vi "Задание_АБ_новые_наработки.vi"() -> ()   [LabVIEW 2017]
uses:
  <vilib>/Analysis/baseanly.llb/Mean (DBL).vi
  <vilib>/gmath/statdist.llb/Beta Random.vi
  <vilib>/Analysis/3filter.llb/Bessel Filter (DBL).vi
  <vilib>/Analysis/NI_AALBase.lvlib
  <vilib>/gmath/NI_Gmath.lvlib
panel:
  out "output array":dbl[](array[numeric])
  out "Array 2":dbl[](array[numeric])
  out "Numeric":i32
  out "Последовательность в массиве":dbl[](array[numeric])
  in  "Кол-во элементов":i32=16
  out "Numeric":dbl
  out "Array":dbl[](array[numeric])
  out "Исходное сообщение":dbl[](array[numeric])
  out "Подготовленный к отправке мажоритарный код":dbl[][](array[numeric])
  out "2-х массив на выходе 3":dbl[][](array[numeric])
  in  "Размер окна":i32=4
  in  "Кол-во копий":i32=5
  out "Шум на основе распределения Рэлея":dbl[](graph)
  out "Итого. кол-во бит":i32
  in  "Пороговое значение":dbl
  out "Демодулированный и отфильтрованный сигнал":dbl[][](graph)
  out "Демодулированный сигнал":i16[](graph)
  in  "Нижняя частота среза":dbl
  in  "Порядок фильтра":i64(slide) scale=0.0..20.0
  in  "Переменная floor(x/y)":i32
  out "Модулирующий сигнал":dbl[](graph)
  out "Частотно модулированный цифровой сигнал":dbl[](graph)
  in  "см. 1.2 Циклов в секунду":i32(slide) scale=4.0..50.0
  in  "Сколько битов брать":i32=4
  out "Радио сигнал с паузами":dbl[](graph)
  in  "Кол-во выборок":i32=400
  out "Массив с паузами":dbl[](array[numeric])
  in  "Количество бит":i32=8
  out "Вырезка из массива":dbl[](array[numeric])
  out "Биты на выходе 1":dbl[](array[numeric])
  # "Демодуляция"
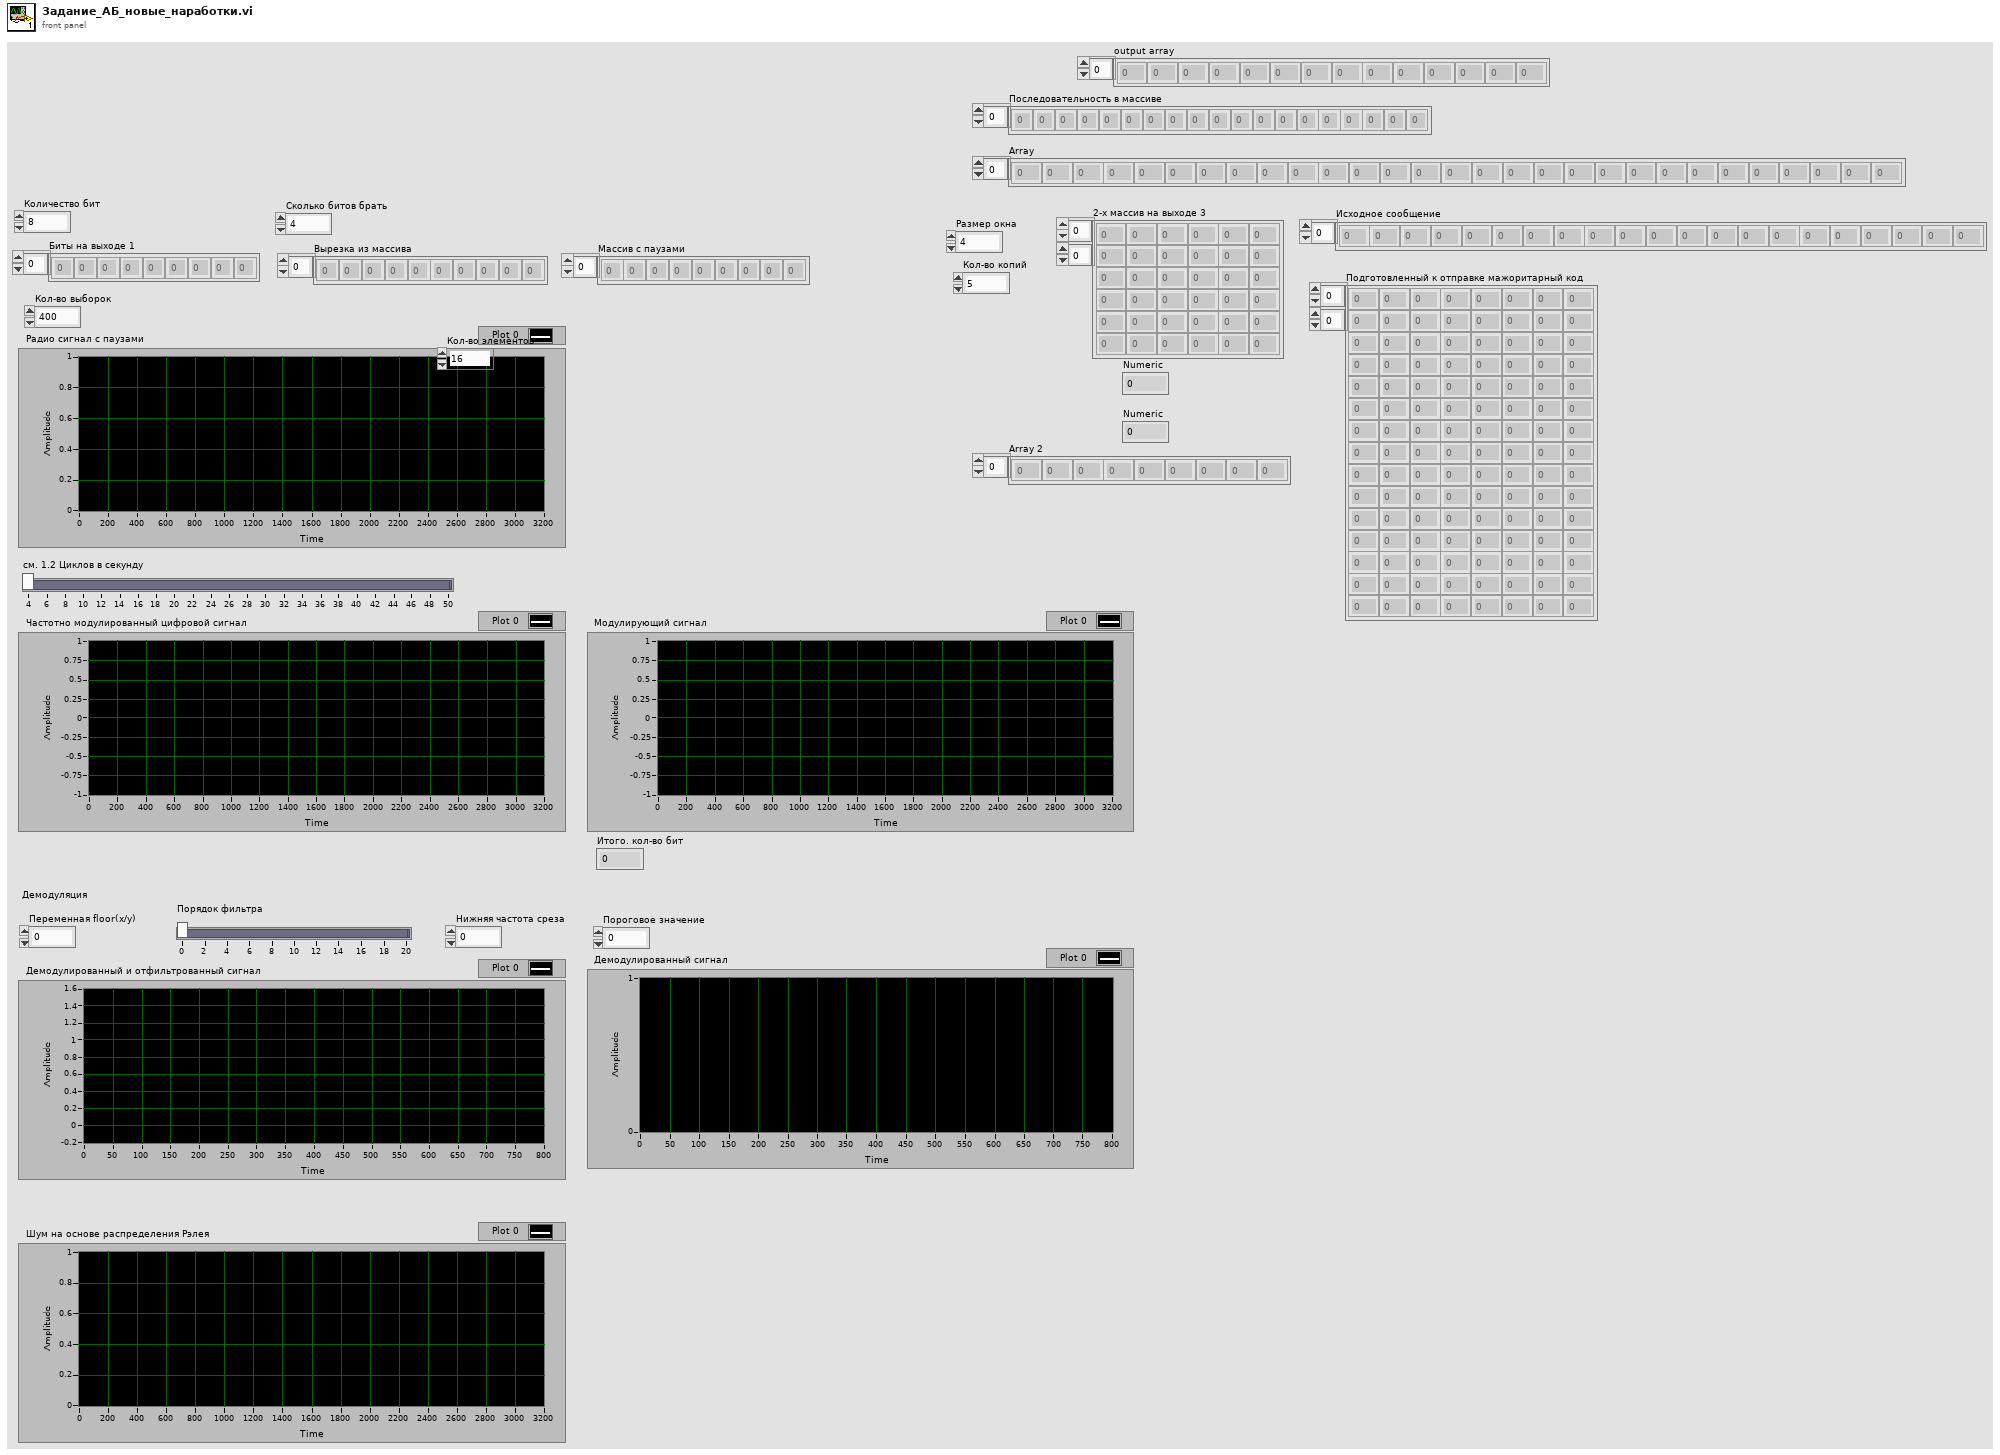
[diagram p1: front panel]
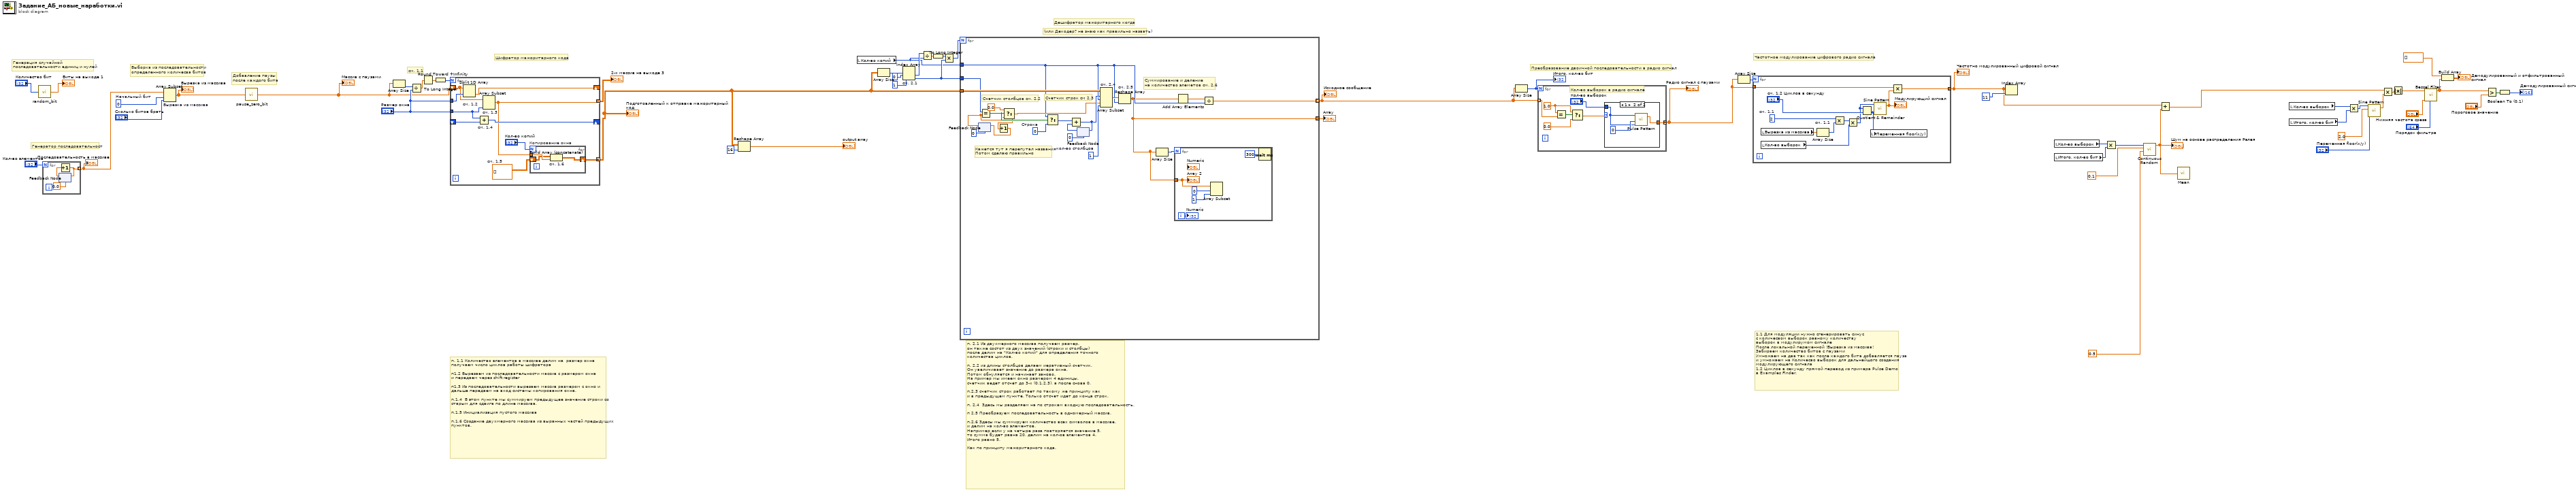
[diagram p0: block diagram]
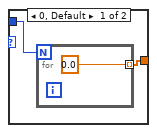
[diagram p2: hidden frame]
diagram:
  w56 = 0  # Начальный бит
  # "Генератор последовательност"
  # "п. 2.1 Из двухмерного массива получаем размер.\nон также состот из двух значений (строки и столбцы) \nпосле делим на \"Кол-во копий\" для определения точного\nколичества циклов.\n\nп. 2.2 из длины столбцов делаем иеративный счетчик. \nОн увеличивает значение до размера окна.\nПотом обнуляется и начинает заново.\nНа пример мы имеем окно размером 4 единицы.\nсчетчик ведет отсчет до 3-х (0,1,2,3), а после снова 0.\n\nп.2.3 счетчик строк работает по такому же принципу как \nи в предыдущем пункте. Только отсчет идет до конца строк.\n\nп. 2.4  Здесь мы разделяем на по строкам входную последовательность.\n\nп 2.5 Преобразуем последовательность в одномерный массив.\n\nп.2.6 Здесы мы суммируем количество всех символов в массиве.\nи делим на кол-во элементов.\nНапример если у на четыре раза повторяется значение 5, \nто сумма будет равна 20, делим на кол-ов элементов 4. \nИтого равно 5. \n\nКак по принципу мажоритарного кода."
  # "см. 1.1"
  # "(или Декодер? не знаю как правильно назвать)"
  # "Дешифратор мажоритарного когда"
  # "п. 1.1 Количество элементов в массиве делим на  размер окна\nполучаем число циклов работы шифратора\n\nп1.2 Вырезаем из последовательности массив с размером окна \nи передаем через shift register\n\nп1.3 Из последовательности вырезаем массив размером с окно и \nдальше передаем на вход системы копирования окна.\n \nп.1.4  В этом пункте мы суммируем предыдущее значение строки со\nстарым для сдвига по длине массива.\n\nп.1.5 Инициализация пустого массива\n\nп.1.6 Создание двухмерного массива из выранных частей предыдущих\nпунктов."
  # "Шифратор мажоритарного кода"
  # "1.1 Для модуляции нужно сгенерировать синус \nс количесвом выборок равному количеству \nвыборок в модулирумом сигнале\nПосле локальной переменной !Вырезка из массива! \nЗабираем количество битов с паузами \nУмножаем на два так как после каждого бита добавляется пауза\nи умножаем на Количесво выборок для дальнейшого создания  \nмодулирующего сигнала\n1.2 Циклов в секунду прямой перевод из примера Pulse Demo \nв Examples Finder."
  # "Преобразование двоичной последовательности в радио сигнал"
  # "Частотное модулирование цифрового радио сигнала"
  # "Добавление паузы \nпосле каждого бита"
  # "Выборка из последовательности\nопределенного количесва битов"
  # "Генерация случайной \nпоследовательности единиц и нулей"
  n1 = call "random_bit.vi"("Количество бит"="Количество бит") -> ("Биты на выходе 1"=→"Биты на выходе 1":dbl[])
  n2 = for {
    N: "Кол-во элементов" -> [_]
    tunnel: [w57] -> w4 mode=indexing
    n3 = feedback #1(0.0) -> (w59:dbl)
    n4 = Increment(x=w59) -> (x+1=w57:dbl)
    n5 = feedback-in #1(w57) -> ()
  }
  "Последовательность в массиве" <- w4
  n6 = Array Subset "Вырезка из массива"(array=w4, index=w56, length="Сколько битов брать") -> (w9:dbl[])
  "Вырезка из массива" <- w9
  n7 = call "pause_zero_bit.vi"("Входная последовательность"=w9) -> ("Массив с паузами"=w8:dbl[])
  "Массив с паузами" <- w8
  n8 = Array Size(array=w8) -> (size(s)=w26:i32)
  n9 = Divide(x=w26, y="Размер окна") -> (x/y=w25:dbl)
  n10 = Round Toward +Infinity(x=w25) -> (ceil(x): smallest int >= x=w24:dbl)
  n11 = To Long Integer(number=w24) -> (32bit integer=w21:i32)
  n12 = for {
    N: w21 -> [_]
    shift-right: [w69] -> _
    shift-left: w8 -> [w67]
    tunnel: "Размер окна" -> [w68]
    shift-right: [w65] -> _
    shift-left: _ -> [w64]
    tunnel: "Размер окна" -> [w66]
    tunnel: [w62] -> w22 mode=indexing
    tunnel: [w61] -> w3 mode=concatenating
    w60 = dbl[][] []  # см. 1.5
    n13 = Split 1D Array "см. 1.2"(array=w67, index=w68) -> (second subarray=w69:dbl[])  [unwired: 1 out]
    n14 = Add "см. 1.4"(x=w66, y=w64) -> (x+y=w65:i32)
    n15 = Array Subset "см. 1.3"(array=w67, length=w66) -> (w62:dbl[])  [unwired: 1 in]
    n16 = for "Копирование окна" {
      N: "Кол-во копий" -> [_]
      tunnel: w62 -> [w71]
      shift-right: [w72] -> w61
      shift-left: w60 -> [w70]
      n17 = Build Array (concatenate) "см. 1.6"(w70, w71) -> (w72:dbl[][])
    }
  }
  "2-х массив на выходе 3" <- w22
  "Подготовленный к отправке мажоритарный код" <- w3
  n18 = Reshape Array(w3, 16 ("dimension size")) -> (→"output array":dbl[])
  n19 = local read "Кол-во копий"() -> (w12:i32)
  n20 = Array Size(array=w3) -> (size(s)=w20:i32[])
  n21 = Index Array "см. 2.1"(array=w20, index #1=0 ("index"), index #2=1 ("index")) -> (element #1=w17:i32, element #2=w16:i32)
  n22 = Divide(x=w17, y=w12) -> (x/y=w15:dbl)
  n23 = To Long Integer(number=w15) -> (32bit integer=w14:i32)
  n24 = Multiply(x=w14, y=w16) -> (x*y=w13:i32)
  n25 = for {
    N: w13 -> [_]
    tunnel: w3 -> [w91]
    tunnel: w16 -> [w84]
    tunnel: w12 -> [w76]
    tunnel: [w75] -> w11 mode=indexing
    tunnel: [w73] -> w7 mode=concatenating
    w90 = 1  # кол-во столбцов
    w82 = 0  # Строка
    # "Суммирование и деление \nна количество элеметов см. 2.6"
    # "Кажется тут я перепутал названия  \nПотом сделаю правильно"
    # "Счетчик строк см 2.3"
    # "Счетчик столбцов см. 2.2"
    n26 = feedback #2(0) -> (w80:dbl)
    n27 = Equal?(x=w84, y=w80) -> (x = y?=w86:bool)
    n28 = Select(t=0.0, s=w86, f=w80) -> (s? t:f=w79:dbl)
    n29 = Increment(x=w79) -> (x+1=w78:dbl)
    n30 = feedback-in #2(w78) -> ()
    n31 = Select(t=w76, s=w86, f=w82) -> (s? t:f=w83:i32)
    n32 = feedback #3(0) -> (w85:i32)
    n33 = Add(x=w83, y=w85) -> (x+y=w81:i32)
    n34 = feedback-in #3(w81) -> ()
    n35 = Array Subset "см. 2.4"(array=w91, index (row)=w81, length (row)=w76, index (col)=w79, length (col)=w90) -> (w92:dbl[][])
    n36 = Reshape Array "см. 2.5"(w92, w76) -> (w73:dbl[])
    n37 = Array Size(array=w73) -> (size(s)=w74:i32)
    n38 = for {
      N: w74 -> [_]
      tunnel: w73 -> [w95]
      i -> [w96]
      n39 = Array Subset(array=w95, index=0, length=1) -> ()  [unwired: 1 out]
      n40 = Wait (ms)(milliseconds to wait=u32 300) -> ()  [unwired: 1 out]
      "Numeric" <- w96
      "Array 2" <- w95
    }
    n41 = Add Array Elements(numeric array=w73) -> (sum=w77:dbl)
    n42 = Divide(x=w77, y=w76) -> (x/y=w75:dbl)
  }
  "Исходное сообщение" <- w11
  "Array" <- w7
  n43 = Array Size(array=w11) -> (size(s)=w53:i32)
  "Итого. кол-во бит" <- w53
  n44 = for {
    N: w53 -> [_]
    tunnel: w11 -> [w101] mode=indexing
    tunnel: [w99] -> w52 mode=concatenating
    w103 = 1.0
    # "Кол-во выборок в радио сигнале"
    n45 = Equal?(x=w103, y=w101) -> (x = y?=w104:bool)
    n46 = Select(t=w103, s=w104, f=0.0) -> (s? t:f=w100:dbl)
    n47 = case shown="1" w100 {
      tunnel: [w105 w109] -> w99
      tunnel: "Кол-во выборок" -> [w106 w108]
      frame 0, Default {
        n48 = for {
          N: w106 -> [_]
          tunnel: [0.0] -> w105 mode=indexing
        }
      }
      frame 1 {
        n49 = call <vilib>:"Pulse Pattern.vi"("width"=w108, "delay"=0, "samples"=w108) -> ("Pulse Pattern"=w109:dbl[])  [unwired: 1 in, 1 out]
      }
    }
  }
  "Радио сигнал с паузами" <- w52
  n50 = Array Size(array=w52) -> (size(s)=w54:i32)
  n51 = for {
    N: w54 -> [_]
    tunnel: w52 -> [w120]
    tunnel: [w119] -> w28
    w115 = 2  # см. 1.1
    n52 = local read "Вырезка из массива"() -> (w117:dbl[])
    n53 = local read "Кол-во выборок"() -> (w113:i32)
    n54 = Array Size "см. 1.1"(array=w117) -> (size(s)=w116:i32)
    n55 = Multiply(x=w115, y=w116) -> (x*y=w114:i32)
    n56 = Multiply(x=w114, y=w113) -> (x*y=w112:i32)
    n57 = Quotient & Remainder(x=w112, y="см. 1.2 Циклов в секунду") -> (floor(x/y)=w111:i32)  [unwired: 1 out]
    n58 = local write "Переменная floor(x/y)"(w111) -> ()
    n59 = call <vilib>:"Sine Pattern.vi"("cycles"=w111, "samples"=w112) -> ("Sinusoidal Pattern"=w118:dbl[])  [unwired: 2 in, 1 out]
    "Модулирующий сигнал" <- w118
    n60 = Multiply(x=w120, y=w118) -> (x*y=w119:dbl[])
  }
  "Частотно модулированный цифровой сигнал" <- w28
  n61 = Index Array(array=w28, index=11 ("index (row)")) -> ()  [unwired: 1 out]
  n62 = local read "Кол-во выборок"() -> (w32:i32)
  n63 = local read "Итого. кол-во бит"() -> (w31:i32)
  n64 = Multiply(x=w32, y=w31) -> (x*y=w30:i32)
  n65 = call-poly <vilib>:"Continuous Random.vi"("b"=0.5, "a"=0.1 ("x"), "samples"=w30) -> ("beta random data"=w29:dbl[])  [unwired: 7 in, 1 out]
  "Шум на основе распределения Рэлея" <- w29
  n66 = Add(x=w28, y=w29) -> (x+y=w27:dbl[])
  n67 = call-poly <vilib>:"Mean.vi"("X"=w29) -> ()  [unwired: 2 out]
  n68 = local read "Кол-во выборок"() -> (w36:i32)
  n69 = local read "Итого. кол-во бит"() -> (w35:i32)
  n70 = Multiply(x=w36, y=w35) -> (x*y=w37:i32)
  n71 = call <vilib>:"Sine Pattern.vi"("cycles"="Переменная floor(x/y)", "amplitude"=2.0, "samples"=w37) -> ("Sinusoidal Pattern"=w39:dbl[])  [unwired: 1 in, 1 out]
  n72 = Multiply(x=w27, y=w39) -> (x*y=w48:dbl[])
  n73 = Absolute Value(x=w48) -> (abs(x)=w45:dbl[])
  n74 = call-poly <vilib>:"Bessel Filter.vi"("order"="Порядок фильтра", "low cutoff freq: fl"="Нижняя частота среза", "X"=w45) -> ("Filtered X"=w43:dbl[])  [unwired: 5 in, 1 out]
  n75 = Build Array(dbl[] [] ("element"), w43) -> (→"Демодулированный и отфильтрованный сигнал":dbl[][])
  n76 = Greater?(x=w43, y="Пороговое значение") -> (0:w42:bool[])
  n77 = Boolean To (0,1)(Boolean=w42) -> (0, 1=→"Демодулированный сигнал":i16[])
